vi "Add N Aliases.vi"(8 "error in":errorcluster, 10 "alias mappings":T1[](array[typedef]), 11 "endpoint aliases in":T3 format="%.0x") -> (0 "error out":errorcluster, 3 "endpoint aliases out":T3 format="%.0x")   [LabVIEW 2020, in "Routing and Faulting Scripting.lvlib"]
doc: "Creates aliases for multiple endpoints."
uses:
  Routing and Faulting Scripting.lvlib
  <vilib>/NI VeriStand/Custom Device API/Custom Device Item Ref.ctl
  Shared/Alias Mapping.ctl
  Shared/Alias Endpoint.ctl
  <vilib>/NI VeriStand/Custom Device API/Custom Device API.lvlib
  Shared/Routing and Faulting Shared.lvlib
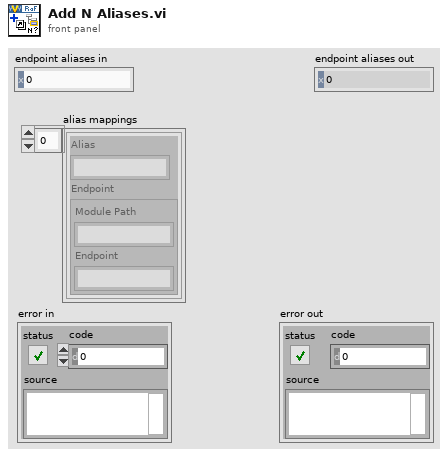
[diagram p1: front panel]
types:
  T1 = typedef "Routing and Faulting Shared.lvlib/Alias Mapping.ctl" = cluster{"Alias":string, "Endpoint":T2}
  T2 = typedef "Routing and Faulting Shared.lvlib/Alias Endpoint.ctl" = cluster{"Module Path":string, "Endpoint":string}
  T3 = typedef "Custom Device API.lvlib/Custom Device Item Ref.ctl" = u64
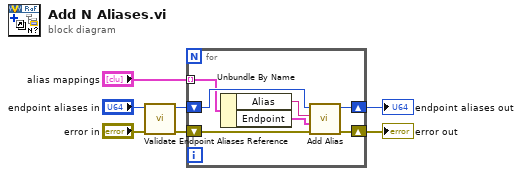
[diagram p0: block diagram]
diagram:
  n1 = call "Validate Endpoint Aliases Reference.vi"("error in"="error in", "endpoint aliases in"="endpoint aliases in") -> ("error out"=w4:errorcluster, "endpoint aliases out"=w2:T3)  [unwired: 8 in]
  n2 = for {
    tunnel: "alias mappings" -> [w12] mode=indexing
    shift-right: [w10] -> w6
    shift-left: w4 -> [w13]
    shift-right: [w9] -> w5
    shift-left: w2 -> [w14]
    n3 = Unbundle By Name(w12) -> ("Alias"=w11:string, "Endpoint"=w8:T2)
    n4 = call "Add Alias.vi"("error in"=w13, "endpoint"=w8, "alias"=w11, "endpoint aliases in"=w14) -> ("error out"=w10:errorcluster, "endpoint aliases out"=w9:T3)  [unwired: 6 in]
  }
  "error out" <- w6
  "endpoint aliases out" <- w5
